vi "writeModeXML.vi"(8 "error in (no error)":errorcluster, 10 "NativeXML in":refnum<class "NativeXML.lvclass">, 11 "PixelflySettings in":refnum<class "PixelflySettings.lvclass">) -> (0 "error out":errorcluster, 2 "NativeXML out":refnum<class "NativeXML.lvclass">, 3 "PixelflySettings out":refnum<class "PixelflySettings.lvclass">)   [LabVIEW 2011, in "Tools.lvlib" / "Settings.lvlib" / "PixelflySettings.lvclass"]
uses:
  PixelflySettings.lvclass
  NativeXML/NativeXML.lvclass
  PixelflySettings.lvclass/PixelflySettings.ctl
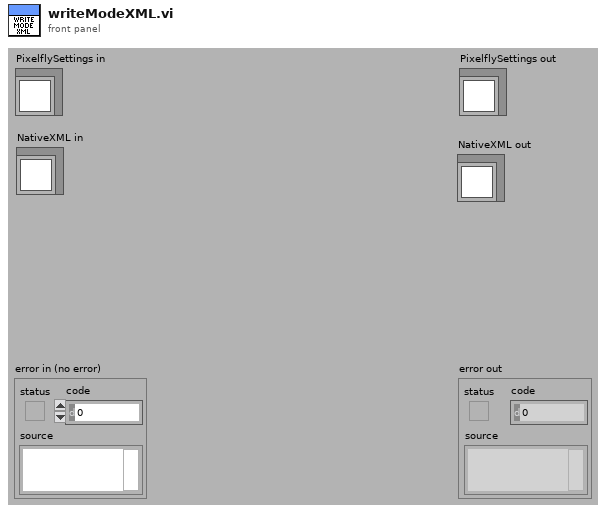
[diagram p1: front panel]
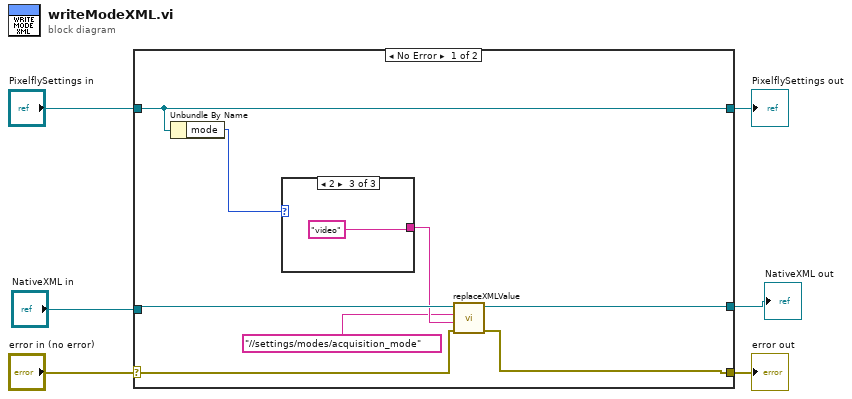
[diagram p0: block diagram]
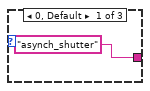
[diagram p2: hidden frame]
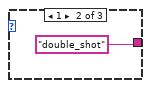
[diagram p3: hidden frame]
diagram:
  n1 = case shown="No Error" "error in (no error)" {
    selector: "error in (no error)" -> [w8 w20]
    tunnel: [w7 w20] -> w5
    tunnel: [w14 w19] -> w3
    tunnel: "PixelflySettings in" -> [w14 w19]
    tunnel: "NativeXML in" -> [w12 w18]
    tunnel: [w11 w18] -> w1
    frame No Error {
      n2 = Unbundle By Name(w14) -> ("mode"=w13:u16)
      n3 = case shown="2" w13 {
        tunnel: ["asynch_shutter" "double_shot" "video"] -> w10
        frame 0, Default {
        }
        frame 1 {
        }
        frame 2 {
        }
      }
      n4 = call "replaceXMLValue.vi"("error in (no error)"=w8, "value"=w10, "replace in"="//settings/modes/acquisition_mode", "NativeXML in"=w12) -> ("error out"=w7:errorcluster, "NativeXML out"=w11:refnum<class "NativeXML.lvclass">)  [unwired: 6 in]
    }
    frame Error {
    }
  }
  "error out" <- w5
  "PixelflySettings out" <- w3
  "NativeXML out" <- w1
